vi "Delete Waypoint Marker.vi"(8 "Error In":errorcluster, 11 "index":i32) -> (0 "error out":errorcluster)   [LabVIEW 2014]
uses:
  C:/Robotic Systems/Products/Surveyor/Software/Ground Station/Data/Mapping DLL/GMap.NET.WindowsForms.dll
  Data/Mapping DLL/GMap.NET.WindowsForms.dll
  Reference/SubVI/Main Map Control Refernce.vi
  Reference/SubVI/GMap DLL Refernce.vi
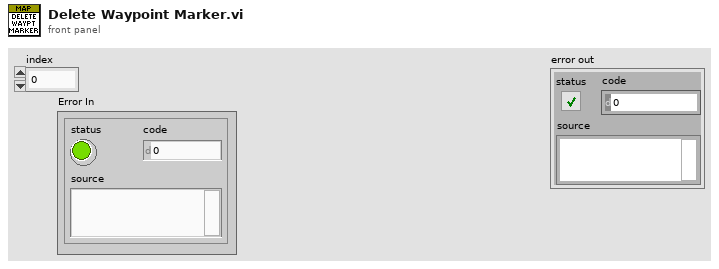
[diagram p1: front panel]
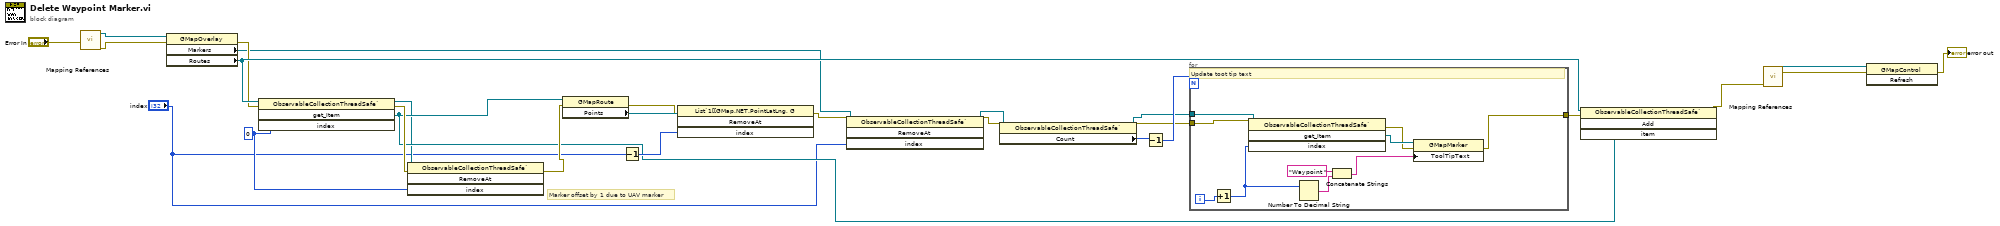
[diagram p0: block diagram]
diagram:
  w21 = 0 ("index")
  # "Marker offset by 1 due to UAV marker"
  n1 = call-poly "Mapping References.vi"("Error In"="Error In") -> ("Error Out"=w26:errorcluster, "Main Map Reference"=w27:refnum<k24>)  [unwired: 9 in]
  n2 = property class="GMapOverlay"(reference=w27, error in=w26) -> (error out=w12:errorcluster, "Markers"=w10:refnum<k24>, "Routes"=w13:refnum<k24>)  [unwired: 1 out]
  n3 = invoke class="ObservableCollectionThreadSafe`" method="get_Item"(reference=w13, error in=w12, "index"=w21) -> (reference out=w14:refnum<k24>, error out=w17:errorcluster, "get_Item"=w15:refnum<k24>)  [unwired: 1 in, 1 out]
  n4 = invoke class="ObservableCollectionThreadSafe`" method="RemoveAt"(reference=w14, error in=w17, "index"=w21) -> (error out=w20:errorcluster)  [unwired: 1 in, 3 out]
  n5 = property class="GMapRoute"(reference=w15, error in=w20) -> (error out=w11:errorcluster, "Points"=w24:refnum<k24>)  [unwired: 1 out]
  n6 = Decrement(x="index") -> (x-1=w23:i32)
  n7 = invoke class="List`1[[GMap.NET.PointLatLng, G" method="RemoveAt"(reference=w24, error in=w11, "index"=w23) -> (error out=w8:errorcluster)  [unwired: 1 in, 3 out]
  n8 = invoke class="ObservableCollectionThreadSafe`" method="RemoveAt"(reference=w10, error in=w8, "index"="index") -> (reference out=w7:refnum<k24>, error out=w6:errorcluster)  [unwired: 1 in, 2 out]
  n9 = property class="ObservableCollectionThreadSafe`"(reference=w7, error in=w6) -> (reference out=w2:refnum<k24>, error out=w3:errorcluster, "Count"=w5:i32)
  n10 = Decrement(x=w5) -> (x-1=w4:i32)
  n11 = for {
    N: w4 -> [_]
    tunnel: w3 -> [w37]
    tunnel: w2 -> [w36]
    tunnel: [w28] -> w1
    i -> [w33]
    # "Update toot tip text"
    n12 = Increment(x=w33) -> (x+1=w30:i32)
    n13 = invoke class="ObservableCollectionThreadSafe`" method="get_Item"(reference=w36, error in=w37, "index"=w30) -> (error out=w34:errorcluster, "get_Item"=w35:refnum<k24>)  [unwired: 1 in, 2 out]
    n14 = Number To Decimal String(number=w30) -> (decimal integer string=w32:string)  [unwired: 1 in]
    n15 = Concatenate Strings("Waypoint " ("string"), w32) -> (w29:string)
    n16 = property class="GMapMarker"(reference=w35, error in=w34, "ToolTipText"=w29) -> (error out=w28:errorcluster)  [unwired: 1 out]
  }
  n17 = invoke class="ObservableCollectionThreadSafe`" method="Add"(reference=w13, error in=w1, "item"=w15) -> (error out=w16:errorcluster)  [unwired: 1 in, 3 out]
  n18 = call-poly "Mapping References.vi"("Error In"=w16) -> ("Error Out"=w19:errorcluster, "GMap DLL Reference"=w18:refnum<k24>)  [unwired: 9 in]
  n19 = invoke class="GMapControl" method="Refresh"(reference=w18, error in=w19) -> (error out=→"error out":errorcluster)  [unwired: 1 in, 2 out]
